vi "Sequence State.vi"(8 "error in (no error)":errorcluster, 9 "Ready?":bool, 10 "Current Nr.":u16=10, 11 "HIJ Vision Camera App Dialog in":refnum<class "HIJ Vision Camera App Dialog.lvclass">) -> (0 "error out":errorcluster, 3 "HIJ Vision Camera App Dialog out":refnum<class "HIJ Vision Camera App Dialog.lvclass">)   [LabVIEW 2014, in "HIJ Vision Camera App Dialog.lvlib" / "HIJ Vision Camera App Dialog.lvclass"]
uses:
  HIJ Vision Camera App Dialog.lvclass
  HIJ Vision Camera App Dialog.lvclass/HIJ Vision Camera App Dialog.ctl
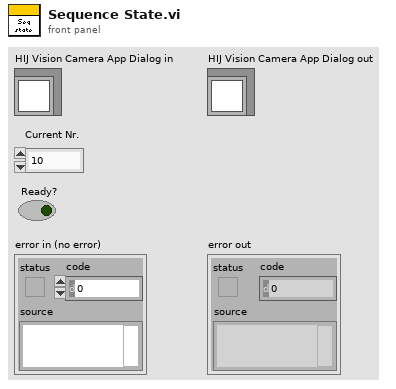
[diagram p1: front panel]
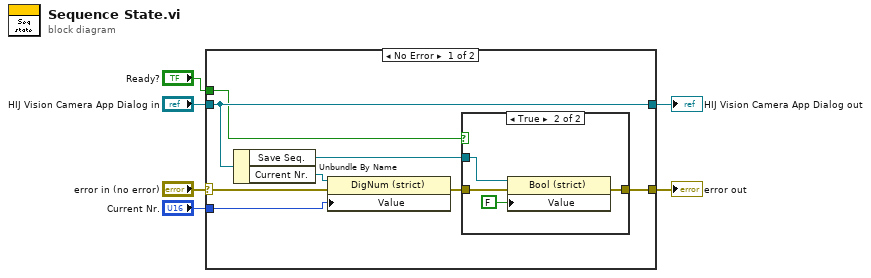
[diagram p0: block diagram]
diagram:
  n1 = case shown="No Error" "error in (no error)" {
    selector: "error in (no error)" -> [w8 w21]
    tunnel: [w7 w21] -> w5
    tunnel: [w14 w20] -> w3
    tunnel: "HIJ Vision Camera App Dialog in" -> [w14 w20]
    tunnel: "Current Nr." -> [w11 _]
    tunnel: "Ready?" -> [w10 _]
    frame No Error {
      n2 = Unbundle By Name(w14) -> ("Save Seq."=w12:refnum<vi>, "Current Nr."=w13:refnum<vi>)
      n3 = property class="DigNum (strict)"(reference=w13, error in=w8, "Value"=w11) -> (error out=w9:errorcluster)  [unwired: 1 out]
      n4 = case shown="True" w10 {
        tunnel: w12 -> [_ w19]
        tunnel: w9 -> [w15 w17]
        tunnel: [w15 w16] -> w7
        frame False {
        }
        frame True {
          n5 = property class="Bool (strict)"(reference=w19, error in=w17, "Value"=FALSE) -> (error out=w16:errorcluster)  [unwired: 1 out]
        }
      }
    }
    frame Error {
    }
  }
  "error out" <- w5
  "HIJ Vision Camera App Dialog out" <- w3
